vi "Create Services.vi"(8 "error in (no error)":errorcluster, 11 "gRPC server in":refnum<class "Servicer.lvclass">) -> (0 "error out":errorcluster, 2 "gRPC services out":refnum<class "ServiceBase.lvclass">[](array[class]), 3 "gRPC server out":refnum<class "Servicer.lvclass">)   [LabVIEW 2019, in "Service Template.lvlib"]
uses:
  Service Template.lvlib
  gRPC lv Servicer/Servicer/Servicer.lvclass
  gRPC lv Servicer/ServiceBase/ServiceBase.lvclass
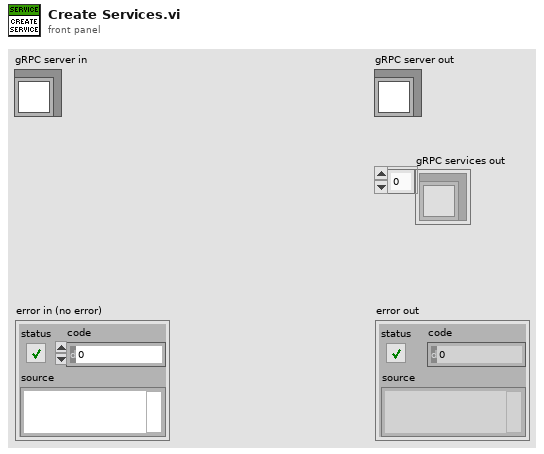
[diagram p1: front panel]
types:
  T1 = typedef "grpc-lvsupport.lvlib/grpcId.ctl" = u64
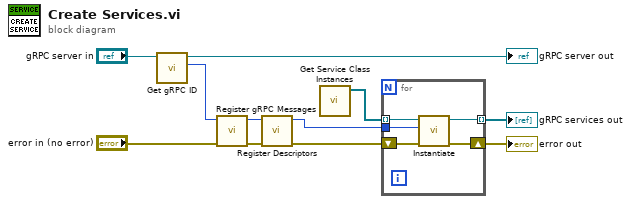
[diagram p0: block diagram]
diagram:
  n1 = call "Get gRPC ID.vi"("gRPC server in"="gRPC server in") -> ("gRPC ID"=w11:T1, "gRPC server out"=→"gRPC server out":refnum<class "Servicer.lvclass">)  [unwired: 9 in]
  n2 = call "Register gRPC Messages.vi"("error in (no error)"="error in (no error)", "gRPC ID"=w11) -> ("error out"=w10:errorcluster, "gRPC ID Out"=w9:T1)  [unwired: 8 in]
  n3 = call "Register Descriptors.vi"("error in (no error)"=w10, "gRPC ID"=w9) -> ("error out"=w7:errorcluster, "gRPC ID Out"=w6:T1)  [unwired: 8 in]
  n4 = call "Get Service Class Instances.vi"() -> ("service instances"=w5:refnum<class "ServiceBase.lvclass">[])  [unwired: 11 in]
  n5 = for {
    tunnel: w6 -> [w14]
    shift-right: [w13] -> w1
    shift-left: w7 -> [w15]
    tunnel: w5 -> [w16] mode=indexing
    tunnel: [w12] -> w2 mode=indexing
    n6 = call-dynamic "Instantiate.vi"("error in"=w15, "gRPCid"=w14, "gRPC service in"=w16) -> ("error out"=w13:errorcluster, "gRPC service out"=w12:refnum<class "ServiceBase.lvclass">)  [unwired: 7 in]
  }
  "error out" <- w1
  "gRPC services out" <- w2
